vi "AI_OpenConfig.vi"(0 "SampleSettings":T3={"samples per channel"=100, "SampleRate"=1000.0, "TansMaxLength"=500000.0, "ReadTimeOut"=10.0, "时钟源"=""}, 1 "AI_ChannelSettings":T1 {"AI_SettingsArry"."标定系数"."Offset" format="%_4g"; "AI_SettingsArry"."标定系数"."Scale" format="%.4g"; "AI_SettingsArry"."shunt resistor location" items=["默认"=-1, "内部"=10200, "外部"=10167]; "AI_SettingsArry"."external shunt resistor value" format="%0.2f"; "AI_SettingsArry"."输入信号类型" items=["默认"=-1, "RSE"=10083, "NRSE"=10078, "差分"=10106, "伪差分"=12529]; "AI_SettingsArry"."单位" items=["安培"=10342, "伏特"=10348, "来自自定义换算"=10065]}, 5 "error in":errorcluster caption="错误输入", 6 "DAQ_AI_task_out":refnum<k21>) -> (14 "DAQ_AI_task_out":refnum<k21>, 19 "error out":errorcluster caption="错误输出")   [LabVIEW 2020, in "DAQ.lvlib" / "NI_DAQ.lvclass"]
uses:
  NI_DAQ.lvclass
  DAQ_Base_class/protected/SampleSettings.ctl
  DAQ_Base_class/protected/AI_ChannelSettings.ctl
  <vilib>/DAQmx/create/channels.llb/DAQmx Create Channel (AI-Voltage-Basic).vi
  <vilib>/DAQmx/create/channels.llb/DAQmx Create Channel (AI-Current-Basic).vi
  <vilib>/DAQmx/configure/timing.llb/DAQmx Timing (Sample Clock).vi
  DAQ_Base_class/DAQ_Base.lvclass
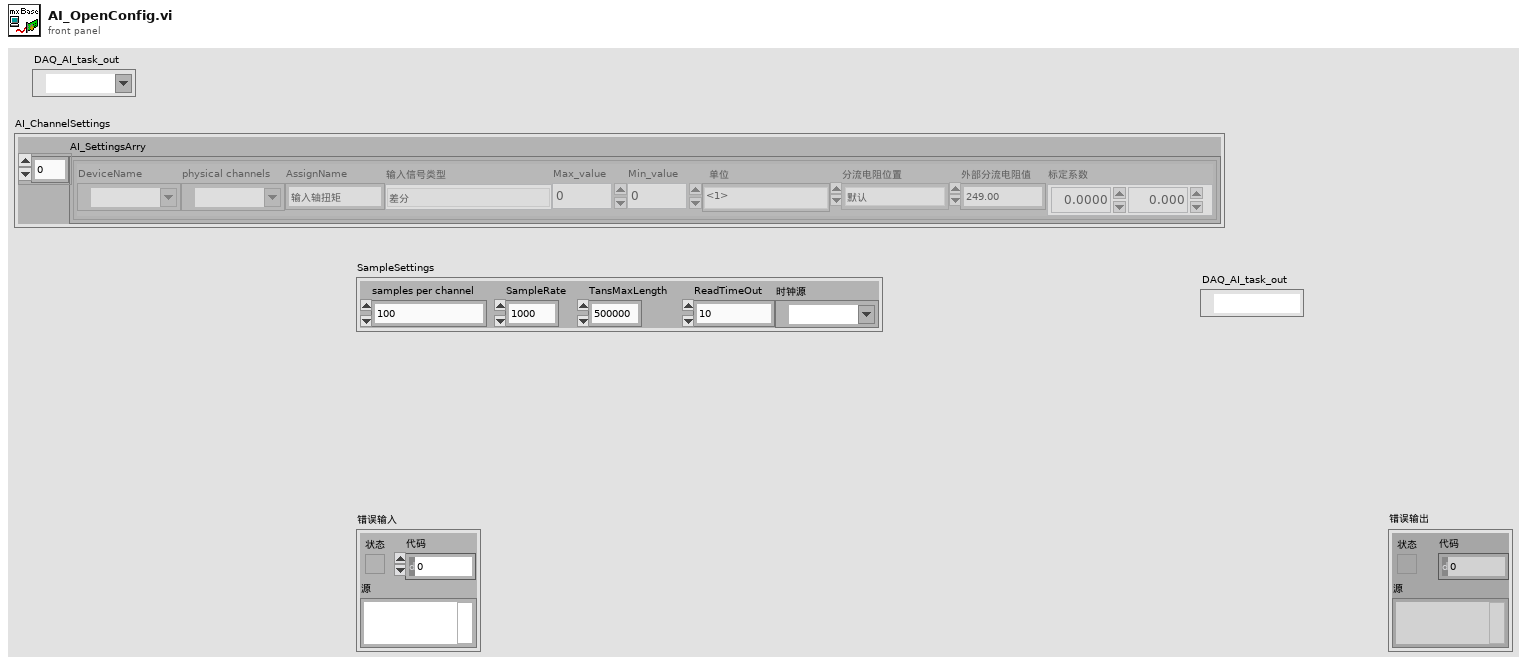
[diagram p1: front panel]
types:
  T1 = typedef "DAQ.lvlib/DAQ_Base.lvclass/AI_ChannelSettings.ctl" = cluster{"AI_SettingsArry":cluster{"DeviceName":tag, "physical channels":tag, "AssignName":string, "输入信号类型":T2, "Max_value":dbl, "Min_value":dbl, "单位":i32, "shunt resistor location":i32, "external shunt resistor value":dbl, "标定系数":cluster{"Scale":dbl, "Offset":dbl}}[]}
  T2 = typedef "AI信号类型.ctl" = i32
  T3 = typedef "DAQ.lvlib/DAQ_Base.lvclass/SampleSettings.ctl" = cluster{"samples per channel":i32, "SampleRate":dbl, "TansMaxLength":dbl, "ReadTimeOut":dbl, "时钟源":tag}
  T4 = cluster{"DeviceName":tag, "physical channels":tag, "AssignName":string, "输入信号类型":T2, "Max_value":dbl, "Min_value":dbl, "单位":i32, "shunt resistor location":i32, "external shunt resistor value":dbl, "标定系数":cluster{"Scale":dbl, "Offset":dbl}}[]
  T5 = cluster{"DeviceName":tag, "physical channels":tag, "AssignName":string, "输入信号类型":T2, "Max_value":dbl, "Min_value":dbl, "单位":i32, "shunt resistor location":i32, "external shunt resistor value":dbl, "标定系数":cluster{"Scale":dbl, "Offset":dbl}}
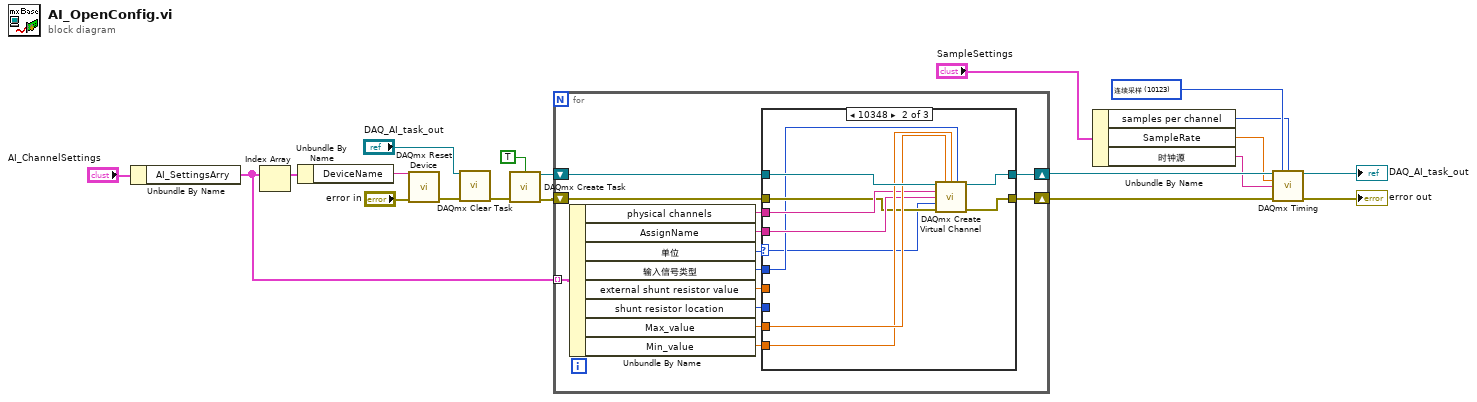
[diagram p0: block diagram]
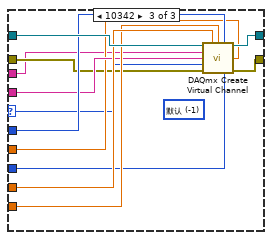
[diagram p3: hidden frame]
diagram:
  w18 = 10123 items=["有限采样"=10178, "连续采样"=10123, "硬件定时单点"=12522] ("sample mode")
  n1 = Unbundle By Name("AI_ChannelSettings") -> ("AI_SettingsArry"=w5:T4)
  n2 = Index Array(array=w5) -> (element=w13:T5)  [unwired: 1 in]
  n3 = Unbundle By Name(w13) -> ("DeviceName"=w12:tag)
  n4 = call <vilib>:"DAQmx Reset Device.vi"("device in"=w12, "error in"="error in") -> ("error out"=w3:errorcluster)  [unwired: 13 in]
  n5 = call <vilib>:"DAQmx Clear Task.vi"("task in"="DAQ_AI_task_out", "error in"=w3) -> ("error out"=w2:errorcluster)  [unwired: 13 in]
  n6 = call <vilib>:"DAQmx Create Task.vi"("auto cleanup"=TRUE, "error in"=w2) -> ("task out"=w17:refnum<k21>, "error out"=w16:errorcluster)  [unwired: 3 in, 9 out]
  n7 = for {
    tunnel: w5 -> [w33] mode=indexing
    shift-right: [w30] -> w20
    shift-left: w17 -> [w31]
    shift-right: [w23] -> w19
    shift-left: w16 -> [w22]
    n8 = Unbundle By Name(w33) -> ("physical channels"=w32:tag, "AssignName"=w29:string, "单位"=w21:i32, "输入信号类型"=w28:T2, "external shunt resistor value"=w25:dbl, "shunt resistor location"=w24:i32, "Max_value"=w27:dbl, "Min_value"=w26:dbl)
    n9 = case shown="10348" w21 {
      selector: w21 -> [_ w36 w47]
      tunnel: w32 -> [_ w41 w48]
      tunnel: w31 -> [w35 w45 w57]
      tunnel: [w35 w44 w56] -> w30
      tunnel: w29 -> [_ w40 w52]
      tunnel: w28 -> [_ w37 w53]
      tunnel: w27 -> [_ w43 w55]
      tunnel: w26 -> [_ w42 w54]
      tunnel: w25 -> [_ _ w51]
      tunnel: w24 -> [_ _ w46]
      tunnel: [w34 w39 w49] -> w23
      tunnel: w22 -> [w34 w38 w50]
      frame Default {
      }
      frame 10348 {
        n10 = call-poly <vilib>:"DAQmx Create Virtual Channel.vi"("task in"=w45, "maximum value"=w43, "minimum value"=w42, "input terminal configuration"=w37, "physical channels"=w41, "name to assign"=w40, "units"=w36, "error in"=w38) -> ("task out"=w44:refnum<k21>, "error out"=w39:errorcluster)  [unwired: 6 in]
      }
      frame 10342 {
        (unwired) -1 items=["默认"=-1, "内部"=10200, "外部"=10167] ("shunt resistor location")
        n11 = call-poly <vilib>:"DAQmx Create Virtual Channel.vi"("task in"=w57, "maximum value"=w55, "minimum value"=w54, "input terminal configuration"=w53, "physical channels"=w48, "name to assign"=w52, "external shunt resistor value"=w51, "units"=w47, "error in"=w50, "shunt resistor location"=w46) -> ("task out"=w56:refnum<k21>, "error out"=w49:errorcluster)  [unwired: 4 in]
      }
    }
  }
  n12 = Unbundle By Name("SampleSettings") -> ("samples per channel"=w15:i32, "SampleRate"=w10:dbl, "时钟源"=w7:tag)
  n13 = call-poly <vilib>:"DAQmx Timing.vi"("task/channels in"=w20, "sample mode"=w18, "samples per channel"=w15, "rate"=w10, "source"=w7, "error in"=w19) -> ("task out"=→"DAQ_AI_task_out":refnum<k21>, "error out"=→"error out":errorcluster)  [unwired: 8 in]
